vi "SW_Load_settings_to_main_tab_2.vi"(0 "Settings path in":path, 2 "Researcher name":string="Researcher", 3 "error in (no error)":errorcluster) -> (6 "Settings cluster out":T1={"Defaults"={"Default User"=0.0, "VISA Resource Name "=""}, "Recording and saving"={"Researcher name"="", "Name prefix"="", "Data filtering"=0, "Stop at"=0.0, "\"Stop at\" enabled"=FALSE}, "Geometry"={"Cage diameter, mm"=0, "Starting angle MIDFIELD"=0, "Starting angle BORDER"=0, "Radius, mm CENTER"=0, "Radius, mm MIDFIELD"=0, "N segments MIDFIELD"=0, "N segments BORDER"=0, "R-gap, mm"=0.0, "Bridge swap"=FALSE, "Bridge H. offset"=0.0, "Bridge V. offset"=0.0, "Twisted neck"=FALSE}, "IO parameters"={"SYNC configuration"=0, "IO 1 configuration"=0, "IO 2 configuration"=0, "IO 3 configuration"=0, "IO 4 configuration"=0, "Activate ext. RS-232"=0, "IO inversion config."=0}, "Stimulus presets array"=[{"Event type"=0, "Dur., s"=0.0, "Stim., s"=0.0, "TTL out N"=1, "Set/Clear"=FALSE, "Stim. has been set"=FALSE}, {"Event type"=0, "Dur., s"=0.0, "Stim., s"=0.0, "TTL out N"=1, "Set/Clear"=FALSE, "Stim. has been set"=FALSE}, {"Event type"=0, "Dur., s"=0.0, "Stim., s"=0.0, "TTL out N"=1, "Set/Clear"=FALSE, "Stim. has been set"=FALSE}, {"Event type"=0, "Dur., s"=0.0, "Stim., s"=0.0, "TTL out N"=1, "Set/Clear"=FALSE, "Stim. has been set"=FALSE}, {"Event type"=0, "Dur., s"=0.0, "Stim., s"=0.0, "TTL out N"=1, "Set/Clear"=FALSE, "Stim. has been set"=FALSE}, {"Event type"=0, "Dur., s"=0.0, "Stim., s"=0.0, "TTL out N"=1, "Set/Clear"=FALSE, "Stim. has been set"=FALSE}, {"Event type"=0, "Dur., s"=0.0, "Stim., s"=0.0, "TTL out N"=1, "Set/Clear"=FALSE, "Stim. has been set"=FALSE}, {"Event type"=0, "Dur., s"=0.0, "Stim., s"=0.0, "TTL out N"=1, "Set/Clear"=FALSE, "Stim. has been set"=FALSE}, {"Event type"=0, "Dur., s"=0.0, "Stim., s"=0.0, "TTL out N"=1, "Set/Clear"=FALSE, "Stim. has been set"=FALSE}, {"Event type"=0, "Dur., s"=0.0, "Stim., s"=0.0, "TTL out N"=1, "Set/Clear"=FALSE, "Stim. has been set"=FALSE}, {"Event type"=0, "Dur., s"=0.0, "Stim., s"=0.0, "TTL out N"=1, "Set/Clear"=FALSE, "Stim. has been set"=FALSE}, {"Event type"=0, "Dur., s"=0.0, "Stim., s"=0.0, "TTL out N"=1, "Set/Clear"=FALSE, "Stim. has been set"=FALSE}, {"Event type"=0, "Dur., s"=0.0, "Stim., s"=0.0, "TTL out N"=1, "Set/Clear"=FALSE, "Stim. has been set"=FALSE}, {"Event type"=0, "Dur., s"=0.0, "Stim., s"=0.0, "TTL out N"=1, "Set/Clear"=FALSE, "Stim. has been set"=FALSE}], "Settings loaded OK"=FALSE} {"Stimulus presets array"."Event type" items=["Stay for N seconds"]; "Stimulus presets array"."TTL out N" items=["1"=1, "2"=2, "1+2"=3]; "Geometry"."Cage diameter, mm" scale=0.0..340.0}, 7 "Settings file path":path, 10 "error out":errorcluster={"status"=TRUE, "code"=1, "source"="Dequeue Element in NI_LVConfig.lvlib:Read Value Without Comment.vi->NI_LVConfig.lvlib:Read Key (I32).vi->SW_Load_settings_to_main_tab.vi"})   [LabVIEW 2018]
uses:
  Controls/CTL_Settings_cluster.ctl
  Controls/CTL_Single_stimulus_setting.ctl
  <vilib>/Utility/config.llb/NI_LVConfig.lvlib
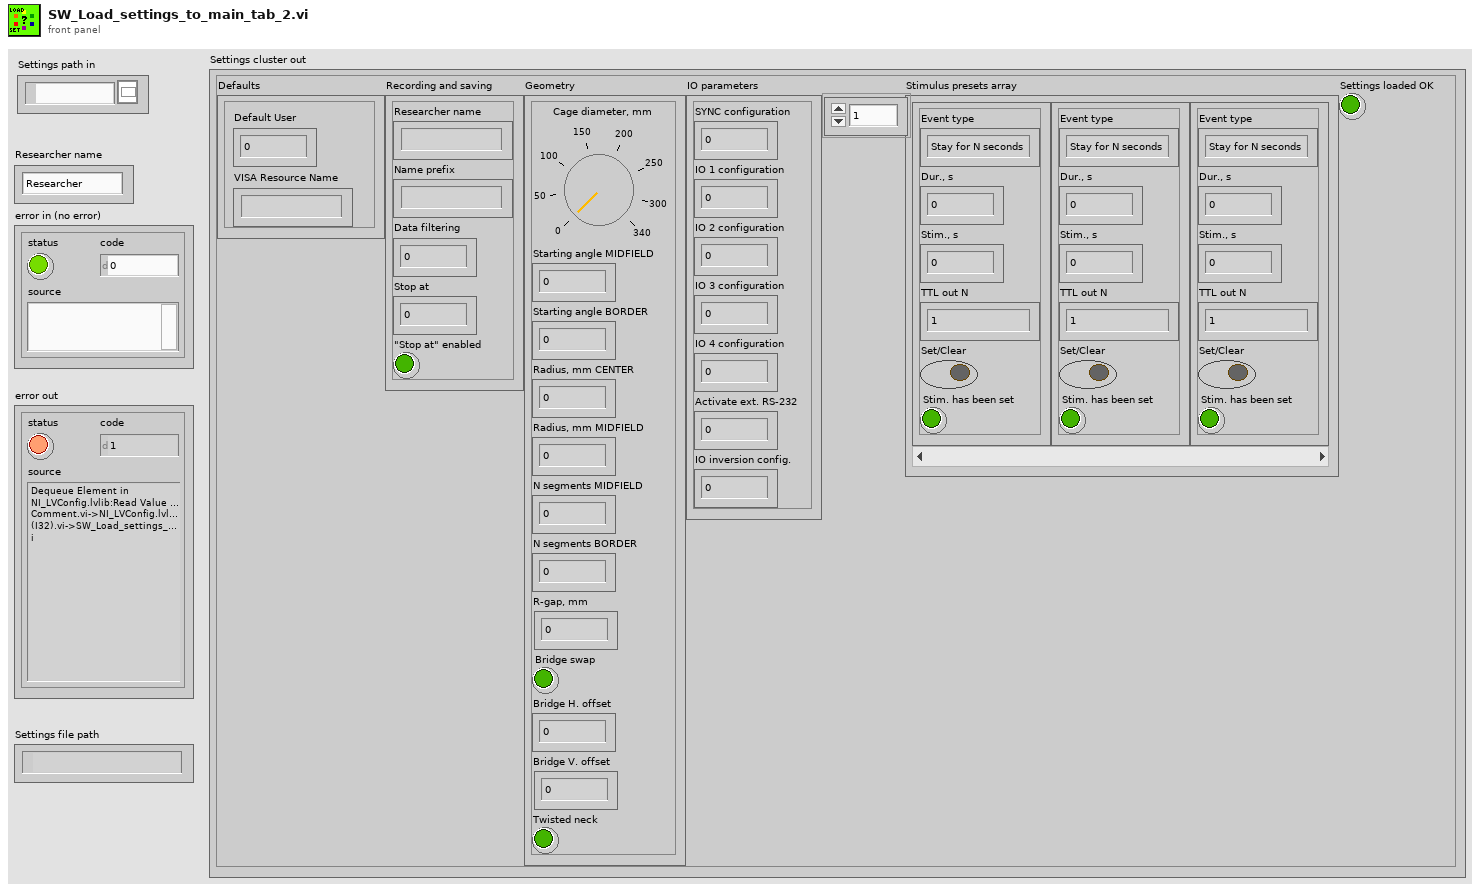
[diagram p1: front panel]
types:
  T1 = typedef "CTL_Settings_cluster.ctl" = cluster{"Defaults":cluster{"Default User":dbl, "VISA Resource Name ":string}, "Recording and saving":cluster{"Researcher name":string, "Name prefix":string, "Data filtering":u16, "Stop at":dbl, "\"Stop at\" enabled":bool}, "Geometry":cluster{"Cage diameter, mm":u16, "Starting angle MIDFIELD":i16, "Starting angle BORDER":i16, "Radius, mm CENTER":u16, "Radius, mm MIDFIELD":u16, "N segments MIDFIELD":u8, "N segments BORDER":u8, "R-gap, mm":sgl, "Bridge swap":bool, "Bridge H. offset":sgl, "Bridge V. offset":sgl, "Twisted neck":bool}, "IO parameters":cluster{"SYNC configuration":u16, "IO 1 configuration":u16, "IO 2 configuration":u16, "IO 3 configuration":u16, "IO 4 configuration":u16, "Activate ext. RS-232":u16, "IO inversion config.":u16}, "Stimulus presets array":T2[], "Settings loaded OK":bool}
  T2 = typedef "CTL_Single_stimulus_setting.ctl" = cluster{"Event type":u16, "Dur., s":sgl, "Stim., s":sgl, "TTL out N":u16, "Set/Clear":bool, "Stim. has been set":bool}
  T3 = typedef "NI_LVConfig.lvlib/Config Data RefNum.ctl" = refnum<k1>
  T4 = cluster{"Default User":dbl, "VISA Resource Name ":string}
  T5 = cluster{"Researcher name":string, "Name prefix":string, "Data filtering":u16, "Stop at":dbl, "\"Stop at\" enabled":bool}
  T6 = cluster{"Cage diameter, mm":u16, "Starting angle MIDFIELD":i16, "Starting angle BORDER":i16, "Radius, mm CENTER":u16, "Radius, mm MIDFIELD":u16, "N segments MIDFIELD":u8, "N segments BORDER":u8, "R-gap, mm":sgl, "Bridge swap":bool, "Bridge H. offset":sgl, "Bridge V. offset":sgl, "Twisted neck":bool}
  T7 = cluster{"SYNC configuration":u16, "IO 1 configuration":u16, "IO 2 configuration":u16, "IO 3 configuration":u16, "IO 4 configuration":u16, "Activate ext. RS-232":u16, "IO inversion config.":u16}
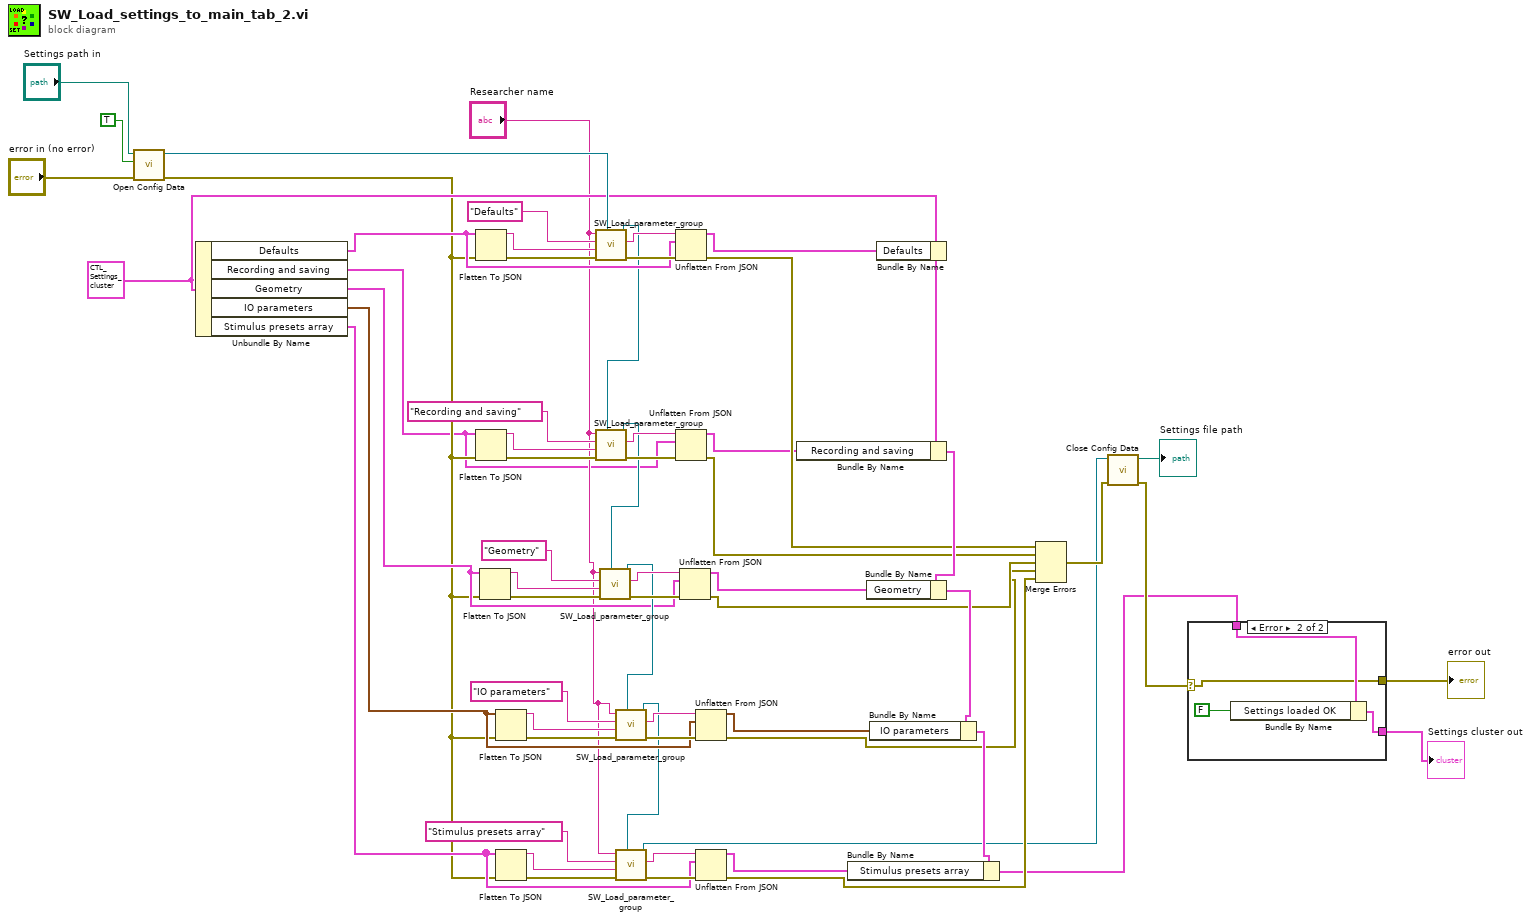
[diagram p0: block diagram]
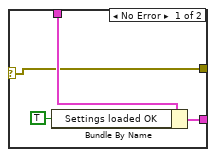
[diagram p2: hidden frame]
diagram:
  w38 = T1 {"Defaults"={"Default User"=0.0, "VISA Resource Name "="Tracker"}, "Recording and saving"={"Researcher name"="Researcher", "Name prefix"="Track", "Data filtering"=5, "Stop at"=0.0, "\"Stop at\" enabled"=FALSE}, "Geometry"={"Cage diameter, mm"=180, "Starting angle MIDFIELD"=0, "Starting angle BORDER"=0, "Radius, mm CENTER"=30, "Radius, mm MIDFIELD"=75, "N segments MIDFIELD"=2, "N segments BORDER"=4, "R-gap, mm"=0.0, "Bridge swap"=FALSE, "Bridge H. offset"=0.0, "Bridge V. offset"=0.0, "Twisted neck"=FALSE}, "IO parameters"={"SYNC configuration"=12, "IO 1 configuration"=1, "IO 2 configuration"=1, "IO 3 configuration"=0, "IO 4 configuration"=0, "Activate ext. RS-232"=0, "IO inversion config."=0}, "Stimulus presets array"=[{"Event type"=0, "Dur., s"=0.0, "Stim., s"=0.0, "TTL out N"=1, "Set/Clear"=FALSE, "Stim. has been set"=FALSE}, {"Event type"=0, "Dur., s"=0.0, "Stim., s"=0.0, "TTL out N"=1, "Set/Clear"=FALSE, "Stim. has been set"=FALSE}, {"Event type"=0, "Dur., s"=0.0, "Stim., s"=0.0, "TTL out N"=1, "Set/Clear"=FALSE, "Stim. has been set"=FALSE}, {"Event type"=0, "Dur., s"=0.0, "Stim., s"=0.0, "TTL out N"=1, "Set/Clear"=FALSE, "Stim. has been set"=FALSE}, {"Event type"=0, "Dur., s"=0.0, "Stim., s"=0.0, "TTL out N"=1, "Set/Clear"=FALSE, "Stim. has been set"=FALSE}, {"Event type"=0, "Dur., s"=0.0, "Stim., s"=0.0, "TTL out N"=1, "Set/Clear"=FALSE, "Stim. has been set"=FALSE}, {"Event type"=0, "Dur., s"=0.0, "Stim., s"=0.0, "TTL out N"=1, "Set/Clear"=FALSE, "Stim. has been set"=FALSE}, {"Event type"=0, "Dur., s"=0.0, "Stim., s"=0.0, "TTL out N"=1, "Set/Clear"=FALSE, "Stim. has been set"=FALSE}, {"Event type"=0, "Dur., s"=0.0, "Stim., s"=0.0, "TTL out N"=1, "Set/Clear"=FALSE, "Stim. has been set"=FALSE}, {"Event type"=0, "Dur., s"=0.0, "Stim., s"=0.0, "TTL out N"=1, "Set/Clear"=FALSE, "Stim. has been set"=FALSE}, {"Event type"=0, "Dur., s"=0.0, "Stim., s"=0.0, "TTL out N"=1, "Set/Clear"=FALSE, "Stim. has been set"=FALSE}, {"Event type"=0, "Dur., s"=0.0, "Stim., s"=0.0, "TTL out N"=1, "Set/Clear"=FALSE, "Stim. has been set"=FALSE}, {"Event type"=0, "Dur., s"=0.0, "Stim., s"=0.0, "TTL out N"=1, "Set/Clear"=FALSE, "Stim. has been set"=FALSE}, {"Event type"=0, "Dur., s"=0.0, "Stim., s"=0.0, "TTL out N"=1, "Set/Clear"=FALSE, "Stim. has been set"=FALSE}], "Settings loaded OK"=FALSE} ("Settings cluster")
  n1 = call <vilib>:"Open Config Data.vi"("error in (no error)"="error in (no error)", "create file if necessary (T)"=TRUE, "configuration file path"="Settings path in") -> ("error out"=w4:errorcluster, "refnum"=w58:T3)  [unwired: 6 in, 1 out]
  n2 = Unbundle By Name(w38) -> ("Defaults"=w53:T4, "Recording and saving"=w3:T5, "Geometry"=w28:T6, "IO parameters"=w27:T7, "Stimulus presets array"=w19:T2[])
  n3 = Flatten To JSON(anything=w53, error in (no error)=w4) -> (JSON string=w57:string, 11:w55:errorcluster)  [unwired: 1 in]
  n4 = Flatten To JSON(anything=w3, error in (no error)=w4) -> (JSON string=w48:string, 11:w50:errorcluster)  [unwired: 1 in]
  n5 = Flatten To JSON(anything=w28, error in (no error)=w4) -> (JSON string=w44:string, 11:w42:errorcluster)  [unwired: 1 in]
  n6 = Flatten To JSON(anything=w27, error in (no error)=w4) -> (JSON string=w31:string, 11:w33:errorcluster)  [unwired: 1 in]
  n7 = Flatten To JSON(anything=w19, error in (no error)=w4) -> (JSON string=w24:string, 11:w22:errorcluster)  [unwired: 1 in]
  n8 = call "SW_Load_parameter_group.vi"("Settings file refnum in"=w58, "error in"=w55, "Default value (JSON)"=w57, "Group"="Defaults", "Researcher name"="Researcher name") -> ("error out"=w59:errorcluster, "Read value (JSON)"=w54:string, "Settings file refnum out"=w46:T3)  [unwired: 4 in]
  n9 = call "SW_Load_parameter_group.vi"("Settings file refnum in"=w46, "error in"=w50, "Default value (JSON)"=w48, "Group"="Recording and saving", "Researcher name"="Researcher name") -> ("error out"=w47:errorcluster, "Read value (JSON)"=w51:string, "Settings file refnum out"=w39:T3)  [unwired: 4 in]
  n10 = call "SW_Load_parameter_group.vi"("Settings file refnum in"=w39, "error in"=w42, "Default value (JSON)"=w44, "Group"="Geometry", "Researcher name"="Researcher name") -> ("error out"=w45:errorcluster, "Read value (JSON)"=w41:string, "Settings file refnum out"=w29:T3)  [unwired: 4 in]
  n11 = call "SW_Load_parameter_group.vi"("Settings file refnum in"=w29, "error in"=w33, "Default value (JSON)"=w31, "Group"="IO parameters", "Researcher name"="Researcher name") -> ("error out"=w30:errorcluster, "Read value (JSON)"=w34:string, "Settings file refnum out"=w17:T3)  [unwired: 4 in]
  n12 = call "SW_Load_parameter_group.vi"("Settings file refnum in"=w17, "error in"=w22, "Default value (JSON)"=w24, "Group"="Stimulus presets array", "Researcher name"="Researcher name") -> ("error out"=w25:errorcluster, "Read value (JSON)"=w21:string, "Settings file refnum out"=w6:T3)  [unwired: 4 in]
  n13 = Unflatten From JSON(JSON string=w54, type and defaults=w53, error in (no error)=w59) -> (value=w52:T4, error out=w16:errorcluster)  [unwired: 4 in]
  n14 = Unflatten From JSON(JSON string=w51, type and defaults=w3, error in (no error)=w47) -> (value=w2:T5, error out=w15:errorcluster)  [unwired: 4 in]
  n15 = Unflatten From JSON(JSON string=w41, type and defaults=w28, error in (no error)=w45) -> (value=w40:T6, error out=w14:errorcluster)  [unwired: 4 in]
  n16 = Unflatten From JSON(JSON string=w34, type and defaults=w27, error in (no error)=w30) -> (value=w35:T7, error out=w13:errorcluster)  [unwired: 4 in]
  n17 = Unflatten From JSON(JSON string=w21, type and defaults=w19, error in (no error)=w25) -> (value=w20:T2[], error out=w12:errorcluster)  [unwired: 4 in]
  n18 = Bundle By Name(cluster=w38, "Defaults"=w52) -> (w37:T1)
  n19 = Bundle By Name(cluster=w37, "Recording and saving"=w2) -> (w36:T1)
  n20 = Bundle By Name(cluster=w36, "Geometry"=w40) -> (w26:T1)
  n21 = Bundle By Name(cluster=w26, "IO parameters"=w35) -> (w18:T1)
  n22 = Bundle By Name(cluster=w18, "Stimulus presets array"=w20) -> (w8:T1)
  n23 = Merge Errors(w16, w15, w14, w13, w12) -> (w11:errorcluster)
  n24 = call <vilib>:"Close Config Data.vi"("error in (no error)"=w11, "refnum"=w6) -> ("error out"=w10:errorcluster, "file path"=→"Settings file path":path)  [unwired: 8 in]
  n25 = case shown="Error" w10 {
    selector: w10 -> [w64 w68]
    tunnel: [w64 w68] -> w9
    tunnel: w8 -> [w66 w70]
    tunnel: [w63 w67] -> w7
    frame No Error {
      n26 = Bundle By Name(cluster=w66, "Settings loaded OK"=TRUE) -> (w63:T1)
    }
    frame Error {
      n27 = Bundle By Name(cluster=w70, "Settings loaded OK"=FALSE) -> (w67:T1)
    }
  }
  "Settings cluster out" <- w7
  "error out" <- w9
